vi "Get Transfer Channels.vi"(8 "error in (no error)":errorcluster, 10 "transfer index":i32, 11 "transfers":T4[](array[typedef]) {"channels"."string offset" format="%d bytes"}) -> (0 "error out":errorcluster, 3 "channels":T1[](array[typedef]) {"string offset" format="%d bytes"})   [LabVIEW 2017, in "DSF Core.lvlib" / "Configuration Session.lvclass"]
doc: "Reads a value associated with a key in a specified section from the configuration data identified by <B>dsf refnum</B>. If the key does not exist, the VI returns the default value. This VI supports multibyte characters in strings. Wire data to the <B>default value</B> input to determine the polymorphic instance to use or manually select the instance."
uses:
  Configuration Session.lvclass
  Typedefs/DSF Engine Transfer Configuration.ctl
  Typedefs/DSF Byte Order.ctl
  Typedefs/DSF Settings Info.ctl
  Typedefs/DSF Engine Channel Configuration.ctl
  Typedefs/DSF Data Type.ctl
  DSF Core.lvlib
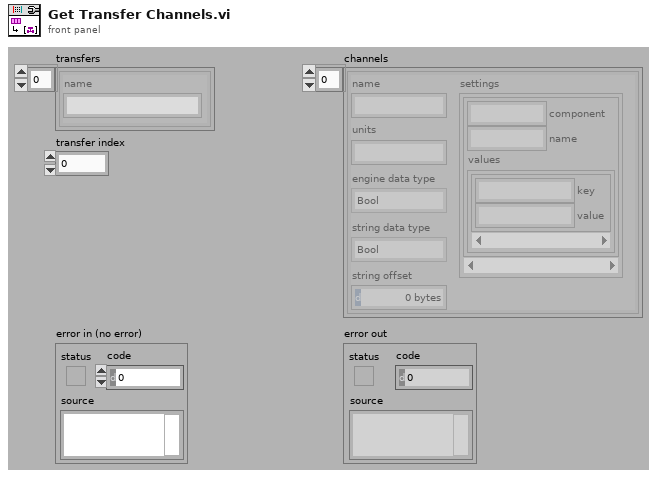
[diagram p1: front panel]
types:
  T1 = typedef "DSF Core.lvlib/DSF Engine Channel Configuration.ctl" = cluster{"string offset":u64, "name":string, "units":string, "engine data type":T2, "string data type":T2, "settings":T3}
  T2 = typedef "DSF Core.lvlib/DSF Data Type.ctl" = enum8{"Bool", "SGL", "DBL", "I8", "I16", "I32", "I64", "U8", "U16", "U32", "U64"}
  T3 = typedef "DSF Core.lvlib/DSF Settings Info.ctl" = cluster{"component":string, "name":string, "values":cluster{"key":string, "value":string}[]}[]
  T4 = typedef "DSF Core.lvlib/DSF Engine Transfer Configuration.ctl" = cluster{"name":string, "byte order":T5, "settings":T3, "channels":T1[]}
  T5 = typedef "DSF Core.lvlib/DSF Byte Order.ctl" = enum8{"big-endian", "little-endian"}
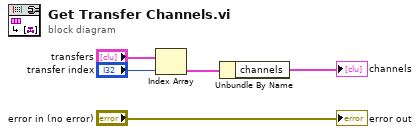
[diagram p0: block diagram]
diagram:
  n1 = Index Array(array="transfers", index="transfer index") -> (element=w2:T4)
  n2 = Unbundle By Name(w2) -> ("channels"=→"channels":T1[])
  "error out" <- "error in (no error)"
